vi "Climb Mode Select.vi"(10 "Set To Manual?":bool, 11 "Set To Auto?":bool) -> (3 "Mode":T1)   [LabVIEW 2015]
uses:
  Common Code/Climb Mode.ctl
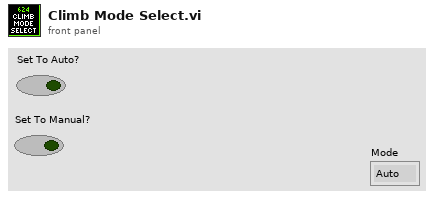
[diagram p1: front panel]
types:
  T1 = typedef "Climb Mode.ctl" = enum16{"Auto", "Manual"}
  T2 = enum16{"0", "1", "2", "3", "4", "5", "6", "7", "8", "9", "A", "B", "C", "D", "E", "F", "G", "H", "I", "J", "K", "L", "M", "N", "O", "P", "Q", "R", "S", "T", "U", "V", "W", "X", "Y", "Z", "F1", "F2", "F3", "F4", "F5", "F6", "F7", "F8", "F9", "F10", "F11", "F12", "F13", "F14", "F15", "ADD", "BACK", "BACKSLASH", "CAPITAL", "COMMA", "DECIMAL", "DELETE", "DIVIDE", "DOWN", "END", "EQUALS", "ESCAPE", "GRAVE (`)", "HOME", "INSERT", "LBRACKET", "LCONTROL", "LEFT", "L ALT", "LSHIFT", "LWIN", "MINUS", "MULTIPLY", "NEXT", "NUMLOCK", "NUMPAD_0", "NUMPAD_1", "NUMPAD_2", "NUMPAD_3", "NUMPAD_4", "NUMPAD_5", "NUMPAD_6", "NUMPAD_7", "NUMPAD_8", "NUMPAD_9", "PAUSE", "PERIOD", "PRIOR (PG UP)", "RBRACKET", "RCONTROL", "RETURN", "RIGHT", "R ALT", "RSHIFT", "RWIN", "SCROLL", "SEMICOLON", "SLASH", "SPACE", "SUBTRACT", "TAB", "UP", "ENTER (num pad)", "' (quote)"}
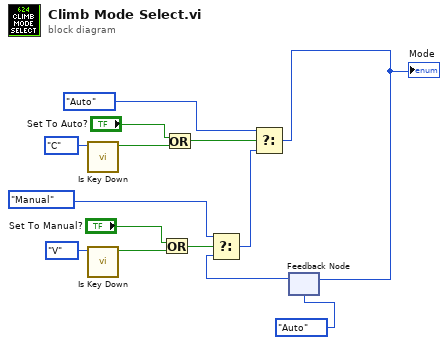
[diagram p0: block diagram]
diagram:
  n1 = call "Is Key Down.vi"("Key"=T2."C") -> ("Key Down?"=w12:bool)  [unwired: 10 in]
  n2 = call "Is Key Down.vi"("Key"=T2."V") -> ("Key Down?"=w8:bool)  [unwired: 10 in]
  n3 = Or(x="Set To Manual?", y=w8) -> (x .or. y?=w7:bool)
  n4 = Or(x="Set To Auto?", y=w12) -> (x .or. y?=w11:bool)
  n5 = feedback #1(Climb_Mode."Auto" ("Mode")) -> (w4:T1)
  n6 = Select(t=Climb_Mode."Manual" ("Mode"), s=w7, f=w4) -> (s? t:f=w5:T1)
  n7 = Select(t=Climb_Mode."Auto" ("Mode"), s=w11, f=w5) -> (s? t:f=w3:T1)
  "Mode" <- w3
  n8 = feedback-in #1(w3) -> ()
